vi "stateChange.vi"(9 "deadZone":dbl, 10 "yTarget":dbl, 11 "xTarget":dbl) -> (3 "targetMet?":bool)   [LabVIEW 2017]
uses:
  TypeDefs/dataFGVState.ctl
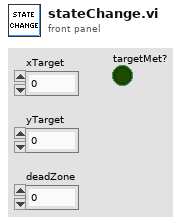
[diagram p1: front panel]
types:
  T1 = typedef "dataFGVState.ctl" = enum16{"init", "write data out", "read data out", "write data in", "read data in"}
  T2 = typedef "dataOut.ctl" = cluster{"X0pos":dbl, "Y0pos":dbl, "Z0pos":dbl, "Fx":dbl, "Fy":dbl, "Fz":dbl, "Encoder1":i32, "Encoder2":i32, "Pot1":dbl, "Pot2":dbl, "Theta0":dbl, "Theta1":dbl, "X1pos":dbl, "Y1pos":dbl, "Z1pos":dbl, "X2pos":dbl, "Y2pos":dbl, "Z2pos":dbl, "ErrorOccurred":bool}
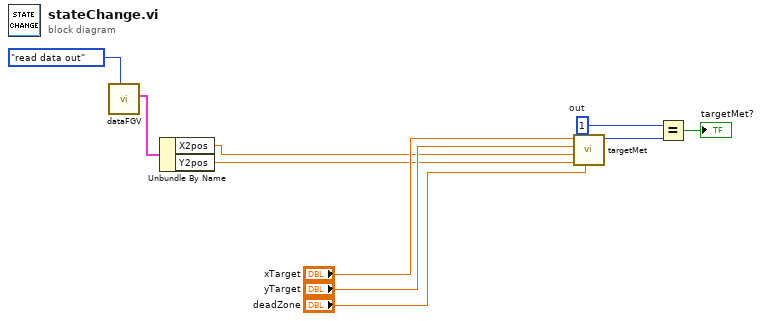
[diagram p0: block diagram]
diagram:
  w3 = 1  # out
  n1 = call "dataFGV.vi"("Enum"=dataFGVState."read data out") -> ("DataOut"=w6:T2)  [unwired: 8 in, 2 out]
  n2 = Unbundle By Name(w6) -> ("X2pos"=w5:dbl, "Y2pos"=w4:dbl)
  n3 = call "targetMet.vi"("Dead Zone (mm)"="deadZone", "Current y (mm)"=w4, "Current x (mm)"=w5, "Target y (mm)"="yTarget", "Target x (mm)"="xTarget") -> ("out"=w2:i32)  [unwired: 6 in]
  n4 = Equal?(x=w3, y=w2) -> (x = y?=→"targetMet?":bool)
